vi "typedefs.vi"   [LabVIEW 2014]
uses:
  modes.ctl
types:
  T1 = typedef "modes.ctl" = enum16{"Initialize", "Up", "Down", "Get User Input"}
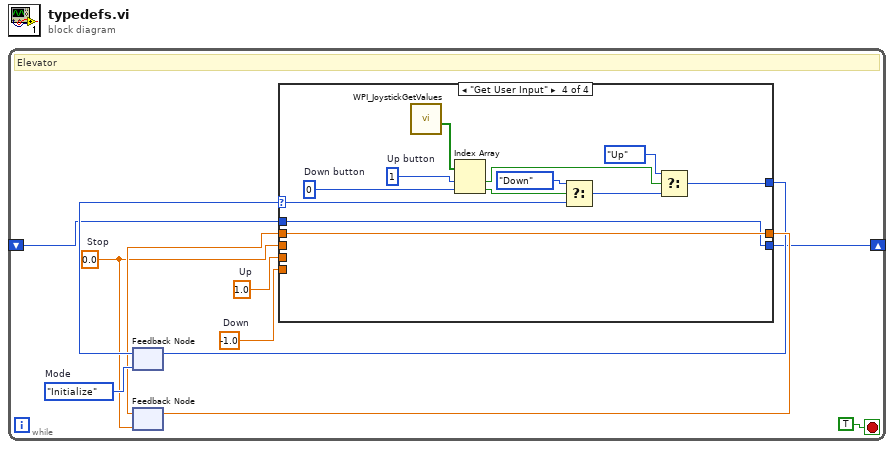
[diagram p0: block diagram]
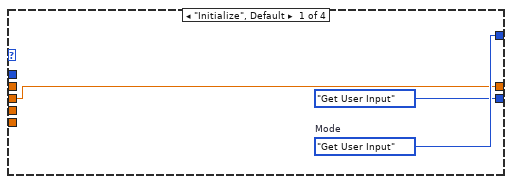
[diagram p2: hidden frame]
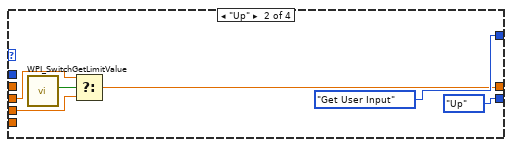
[diagram p3: hidden frame]
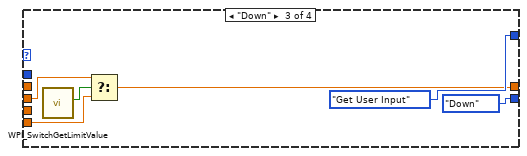
[diagram p4: hidden frame]
diagram:
  n1 = while {
    shift-right: [w2] -> _
    shift-left: _ -> [w1]
    stop <- TRUE stop-if-true
    w5 = 0.0  # Stop
    w8 = -1.0  # Down
    w9 = 1.0  # Up
    w10 = modes."Initialize"  # Mode
    # "Elevator"
    n2 = feedback #1(w10) -> (w11:T1)
    n3 = feedback #2(w5) -> (w6:dbl)
    n4 = case shown="\"Get User Input\"" w11 {
      selector: w11 -> [_ _ _ w36]
      tunnel: [w14 modes."Get User Input" ("Mode") modes."Get User Input" ("Mode") w32] -> w3
      tunnel: w9 -> [_ w18 _ _]
      tunnel: w5 -> [w13 w16 w25 _]
      tunnel: [w13 w17 w22 w28] -> w7
      tunnel: w8 -> [_ _ w24 _]
      tunnel: w6 -> [_ _ _ w28]
      tunnel: [modes."Get User Input" ("Mode") modes."Up" ("Mode") modes."Down" ("Mode") w27] -> w2
      tunnel: w1 -> [_ _ _ w27]
      frame "Initialize", Default {
        w14 = modes."Get User Input"  # Mode
      }
      frame "Up" {
        n5 = call <vilib>:"WPI_SwitchGetLimitValue.vi"() -> ("Switch Pressed"=w20:bool)  [unwired: 9 in, 2 out]
        n6 = Select(t=w16, s=w20, f=w18) -> (s? t:f=w17:dbl)
      }
      frame "Down" {
        n7 = call <vilib>:"WPI_SwitchGetLimitValue.vi"() -> ("Switch Pressed"=w26:bool)  [unwired: 9 in, 2 out]
        n8 = Select(t=w25, s=w26, f=w24) -> (s? t:f=w22:dbl)
      }
      frame "Get User Input" {
        w37 = 0  # Down button
        w38 = 1  # Up button
        n9 = call <vilib>:"WPI_JoystickGetValues.vi"() -> ("Buttons"=w31:bool[])  [unwired: 7 in, 4 out]
        n10 = Index Array(array=w31, index #1=w38, index #2=w37) -> (element #1=w30:bool, element #2=w29:bool)
        n11 = Select(t=modes."Down", s=w29, f=w36) -> (s? t:f=w34:T1)
        n12 = Select(t=modes."Up", s=w30, f=w34) -> (s? t:f=w32:T1)
      }
    }
    n13 = feedback-in #1(w3) -> ()
    n14 = feedback-in #2(w7) -> ()
  }
